vi "Initial Z (SubVI).vi"(2 "error in (no error)":errorcluster, 3 "VISA Refnum in":refnum<visa-resource-name>) -> (0 "error out":errorcluster)   [LabVIEW 2018]
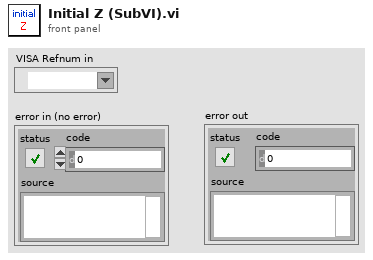
[diagram p1: front panel]
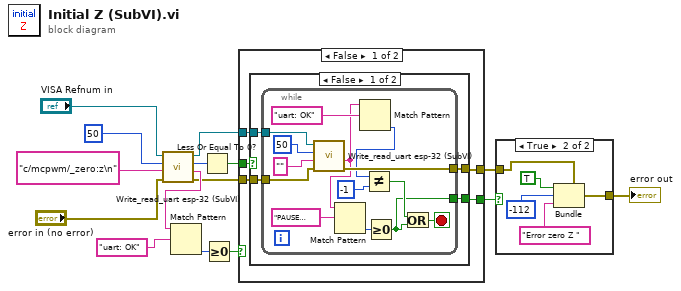
[diagram p0: block diagram]
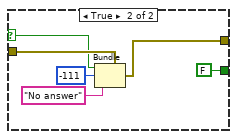
[diagram p2: hidden frame]
diagram:
  n1 = call "Write_read_uart esp-32 (SubVI).vi"("error in (no error)"="error in (no error)", "write buffer"="c/mcpwm/_zero:z\n", "milliseconds to wait"=u32 50, "VISA Refnum in"="VISA Refnum in") -> ("error out 4"=w8:errorcluster, "read buffer"=w9:string, "read bite"=w10:u32, "VISA resource name out"=w11:refnum<visa-resource-name>)
  n2 = Match Pattern(string=w9, regular expression="uart: OK") -> (offset past match=w2:i32)  [unwired: 1 in, 3 out]
  n3 = Less Or Equal To 0?(x=w10) -> (x <= 0?=w12:bool)
  n4 = Greater Or Equal To 0?(x=w2) -> (x >= 0?=w1:bool)
  n5 = case shown="False" w1 {
    tunnel: [w20 w46] -> w15
    tunnel: [w19 w45] -> w14
    tunnel: w12 -> [w18 w45]
    tunnel: w11 -> [w17 _]
    tunnel: w8 -> [w16 w46]
    frame False {
      n6 = case shown="False" w18 {
        selector: w18 -> [_ w42]
        tunnel: w16 -> [w24 w43]
        tunnel: w17 -> [w23 _]
        tunnel: [w22 w39] -> w20
        tunnel: [w21 FALSE] -> w19
        frame False {
          n7 = while {
            tunnel: w24 -> [w36]
            tunnel: w23 -> [w35]
            tunnel: [w31] -> w22
            tunnel: [w25] -> w21
            stop <- w32 stop-if-true
            n8 = call "Write_read_uart esp-32 (SubVI).vi"("error in (no error)"=w36, "write buffer"="", "milliseconds to wait"=u32 50, "VISA Refnum in"=w35) -> ("error out 4"=w31:errorcluster, "read buffer"=w26:string)  [unwired: 2 out]
            n9 = Match Pattern(string=w26, regular expression="PAUSE rotate") -> (offset past match=w27:i32)  [unwired: 1 in, 3 out]
            n10 = Match Pattern(string=w26, regular expression="uart: OK") -> (offset past match=w30:i32)  [unwired: 1 in, 3 out]
            n11 = Not Equal?(x=w30, y=-1 ("offset past match")) -> (x != y?=w29:bool)
            n12 = Greater Or Equal To 0?(x=w27) -> (x >= 0?=w25:bool)
            n13 = Or(x=w29, y=w25) -> (x .or. y?=w32:bool)
          }
        }
        frame True {
          n14 = Bundle(cluster=w43, "status"=w42, "code"=-111, "source"="No answer") -> (w39:errorcluster)
        }
      }
    }
    frame True {
    }
  }
  n15 = case shown="True" w14 {
    tunnel: w15 -> [w47 w51]
    tunnel: [w47 w48] -> w13
    frame False {
    }
    frame True {
      n16 = Bundle(cluster=w51, "status"=TRUE, "code"=-112, "source"="Error zero Z ") -> (w48:errorcluster)
    }
  }
  "error out" <- w13
